vi "UpdateGraphLegends.vi"(9 "Display":T1, 11 "Graph_refs":T2) -> (3 "Graph_refs out":T2)   [LabVIEW 2018]
uses:
  controls/Graph_references.ctl
  controls/graph_controls.ctl
  controls/Data_calc_mode.ctl
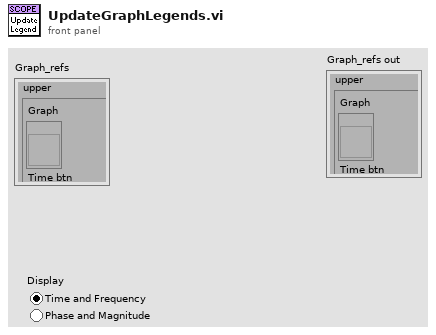
[diagram p1: front panel]
types:
  T1 = typedef "Data_calc_mode.ctl" = enum32{"Time and Frequency", "Phase and Magnitude"}
  T2 = typedef "Graph_references.ctl" = cluster{"upper":T3, "lower":T3, "Freq graph":refnum<vi>, "Adaptive FF graph":refnum<vi>}
  T3 = typedef "graph_controls.ctl" = cluster{"Graph":refnum<vi>, "Time btn":refnum<vi>, "Amplitude btn":refnum<vi>, "Chart":refnum<vi>}
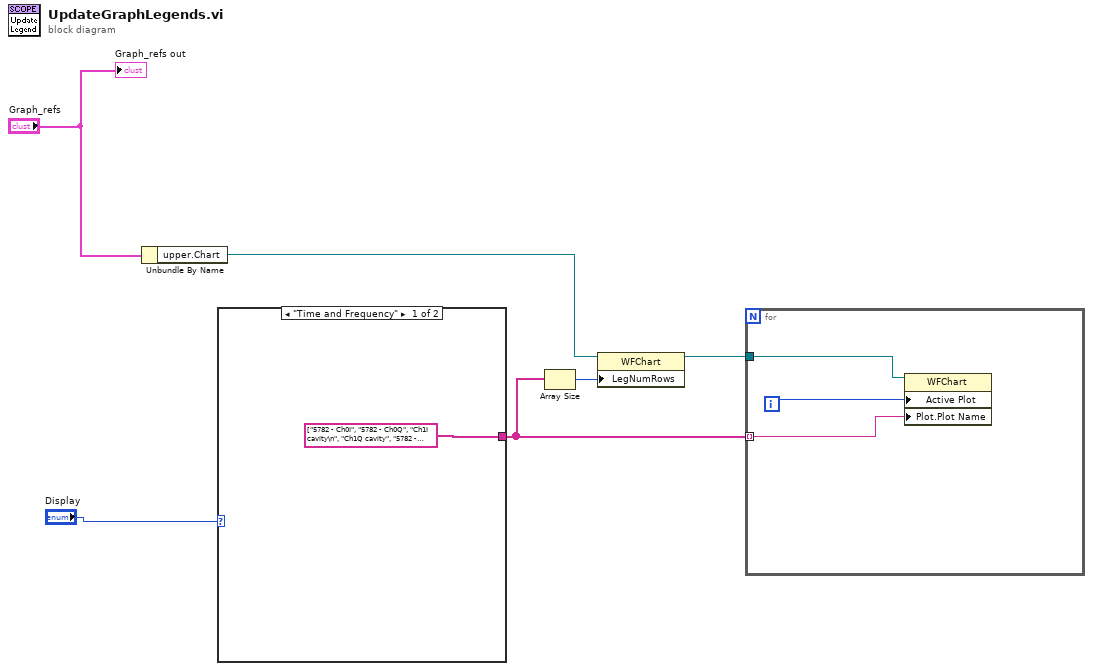
[diagram p0: block diagram]
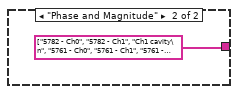
[diagram p2: hidden frame]
diagram:
  n1 = Unbundle By Name("Graph_refs") -> ("upper.Chart"=w5:refnum<vi>)
  n2 = case shown="\"Time and Frequency\"" "Display" {
    tunnel: [string[] ["5782 - Ch0I", "5782 - Ch0Q", "Ch1I cavity\n", "Ch1Q cavity", "5782 - Ch1I", "5782 - Ch1Q", "5761 - Ch0I", "5761 - Ch0Q", "5761 - Ch1I", "5761 - Ch1Q", "5761 - Ch2I", "5761 - Ch2Q"] ("Array") string[] ["5782 - Ch0", "5782 - Ch1", "Ch1 cavity\n", "5761 - Ch0", "5761 - Ch1", "5761 - Ch2", "5761 - Ch3"] ("Array")] -> w2
    frame "Time and Frequency" {
    }
    frame "Phase and Magnitude" {
    }
  }
  n3 = Array Size(array=w2) -> (size(s)=w3:i32)
  n4 = property class="WFChart"(reference=w5, "LegNumRows"=w3) -> (reference out=w1:refnum<vi>)  [unwired: 1 in, 1 out]
  n5 = for {
    tunnel: w2 -> [w10] mode=indexing
    tunnel: w1 -> [w9]
    i -> [w11]
    n6 = property class="WFChart"(reference=w9, "Active Plot"=w11, "Plot.Plot Name"=w10) -> ()  [unwired: 1 in, 2 out]
  }
  "Graph_refs out" <- "Graph_refs"
